vi "题目7.vi"() -> ()   [LabVIEW 2017]
uses:
  <vilib>/Utility/file.llb/Read Delimited Spreadsheet (DBL).vi
  <vilib>/Analysis/NI_AALBase.lvlib
panel:
  in  "周期":dbl
  out "波形图表":dbl[][](graph)
  out "all rows":dbl[][](array[numeric]) caption="所有行"
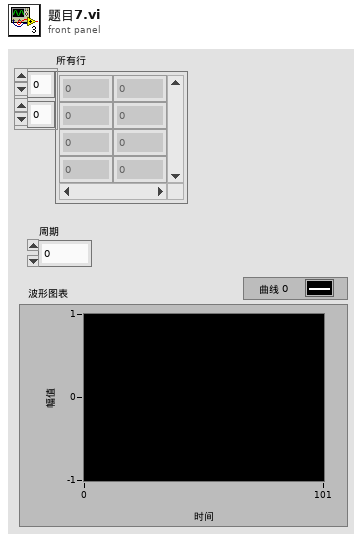
[diagram p1: front panel]
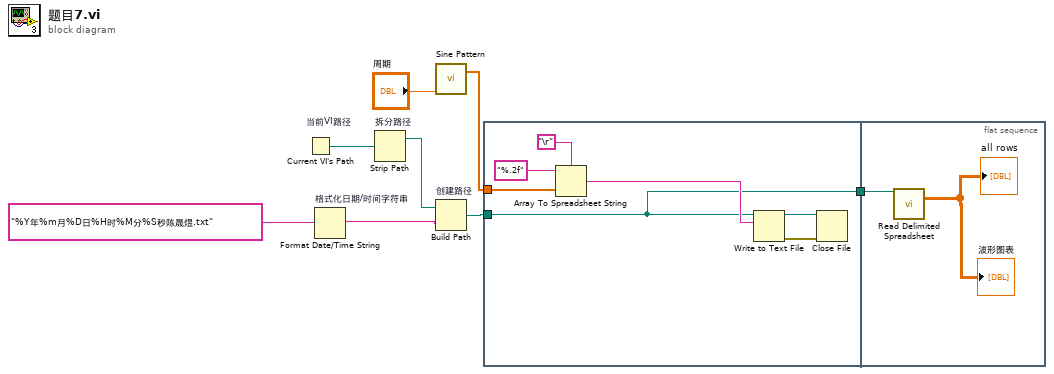
[diagram p0: block diagram]
diagram:
  n1 = Current VI's Path "当前VI路径"() -> (path=w8:path)
  n2 = Format Date/Time String "格式化日期/时间字符串"(time format string (%c)="%Y年%m月%D日%H时%M分%S秒陈晟煜.txt") -> (date/time string=w1:string)  [unwired: 2 in]
  n3 = Strip Path "拆分路径"(path=w8) -> (stripped path=w7:path)  [unwired: 1 out]
  n4 = call <vilib>:"Sine Pattern.vi"("cycles"="周期") -> ("Sinusoidal Pattern"=w4:dbl[])  [unwired: 3 in, 1 out]
  n5 = Build Path "创建路径"(base path=w7, name or relative path=w1) -> (appended path=w5:path)
  n6 = flat-sequence {
    tunnel: w5 -> [w9]
    tunnel: w4 -> [w13]
    tunnel: [w9] -> w3
    tunnel: w3 -> [w17]
    frame #0 {
      n7 = Array To Spreadsheet String(delimiter (Tab)="\r", array=w13, 3:"%.2f" ("格式字符串")) -> (spreadsheet string=w12:string)
      n8 = Write to Text File(file (use dialog)=w9, text=w12) -> (refnum out=w14:refnum<file>, error out=w15:errorcluster)  [unwired: 2 in, 1 out]
      n9 = Close File(refnum=w14, error in=w15) -> ()  [unwired: 2 out]
    }
    frame #1 {
      n10 = call-poly <vilib>:"Read Delimited Spreadsheet.vi"("file path (dialog if empty)"=w17) -> ("all rows"=→"all rows" →"波形图表":dbl[][])  [unwired: 9 in, 5 out]
    }
  }
